vi "测试配置文件生成.vi"() -> ()   [LabVIEW 2013]
uses:
  <vilib>/Utility/config.llb/Write Key (String).vi
  <vilib>/Utility/config.llb/NI_LVConfig.lvlib
panel:
  in  "配置文件全名":path
  in  "写入至从板号":dbl=1.0 min=1.0 max=30.0
  in  "BCU合成程序全名-用于仿真器刷写":path
  in  "BMU应用程序全名":string[][](table)
  in  "更新至指定BMU号":bool
  in  "BMU应用程序全名":path
  in  "配置到全部BMU":bool
  in  "BMU个数":dbl
  in  "BCU应用程序全名-用于在线更新程序":path
  in  "充电CAN波特率":enum16{"250K", "500K"}(ring)
  in  "整车CAN波特率":enum16{"250K", "500K"}(ring)
  in  "内部CAN波特率":enum16{"250K", "500K"}(ring)
  out "取消":bool
  out "确定并启动":bool
  in  "自适就CAN卡类型":bool=TRUE
  in  "退出":bool
  in  "保存":bool
  in  "error in":errorcluster caption="错误输入"
  in  "BMU合成程序全名-用于仿真器刷写":path
  # "自动化测试配置文件生成器"
  # "将BMU应用程序全名："
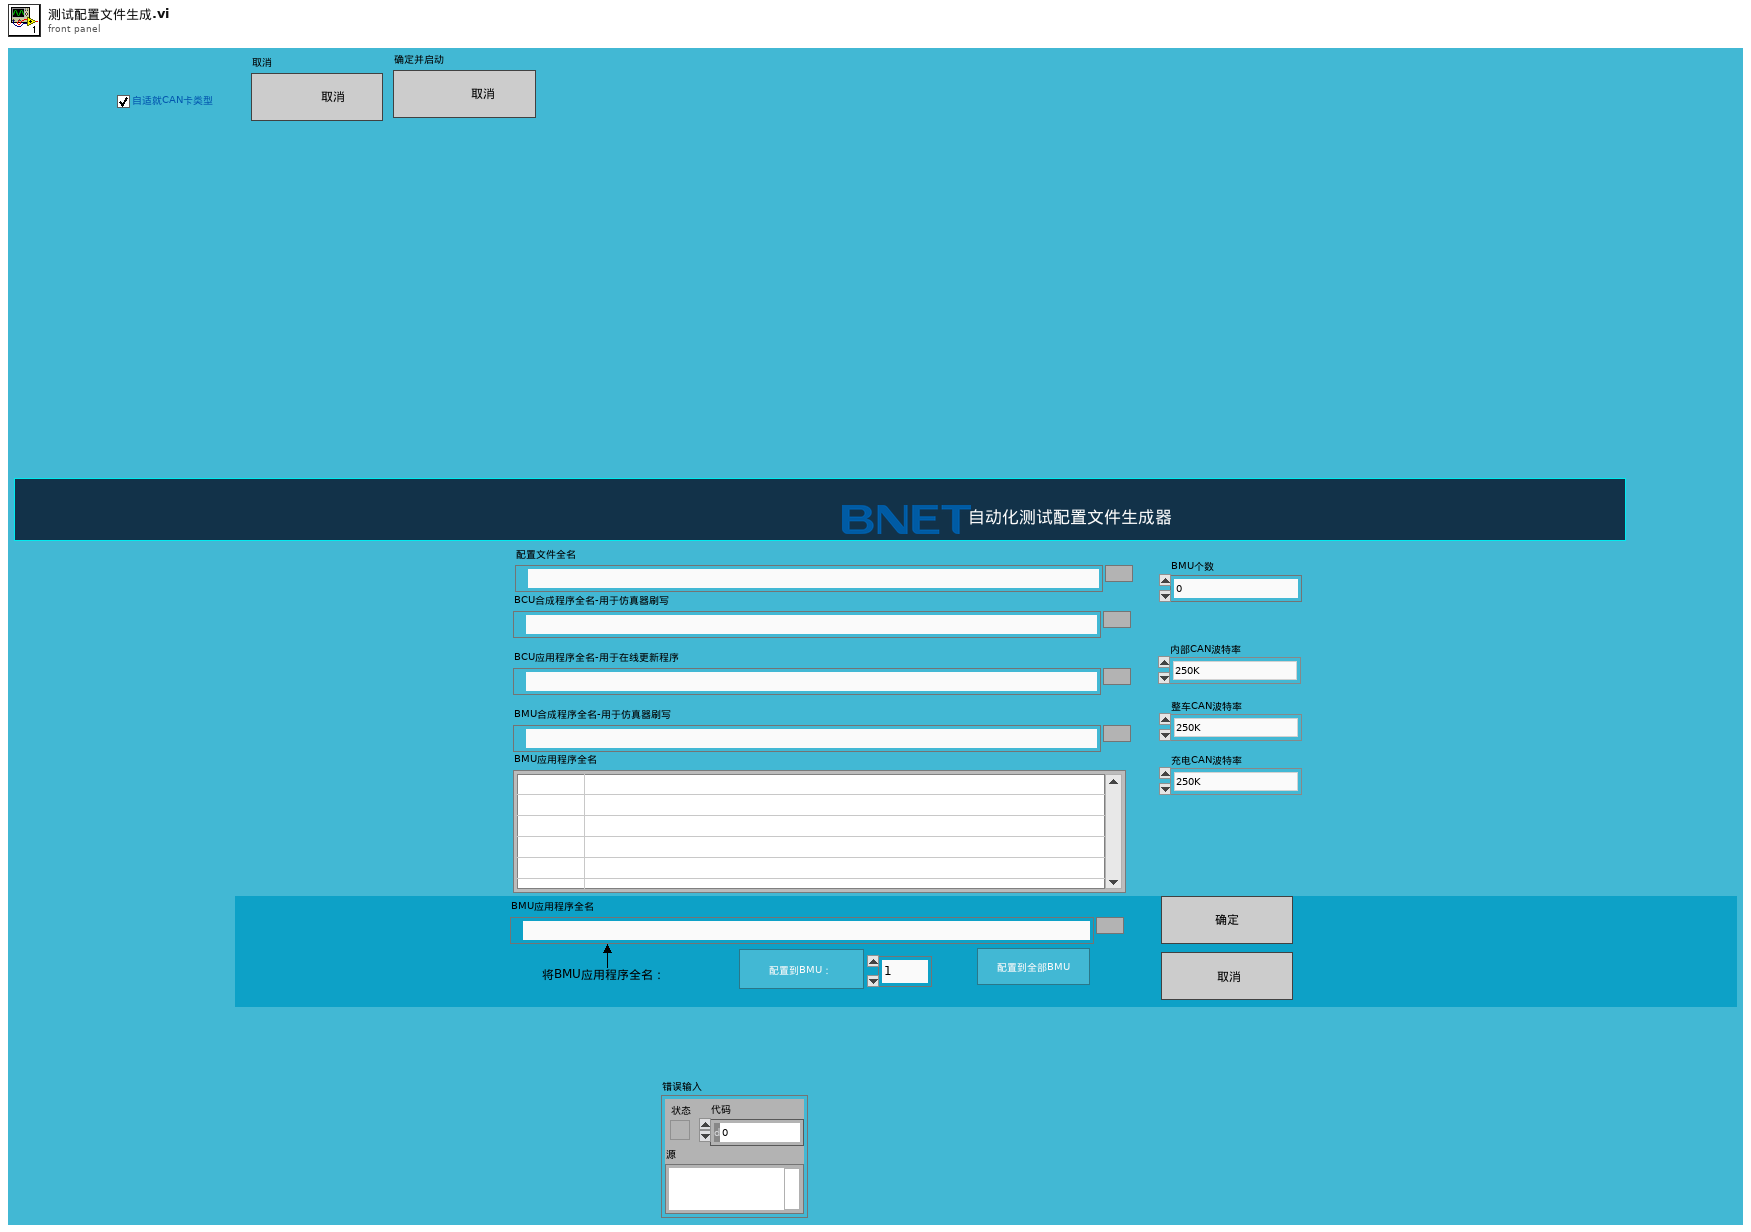
[diagram p1: front panel]
types:
  T1 = typedef "NI_LVConfig.lvlib/Config Data RefNum.ctl" = refnum<k1>
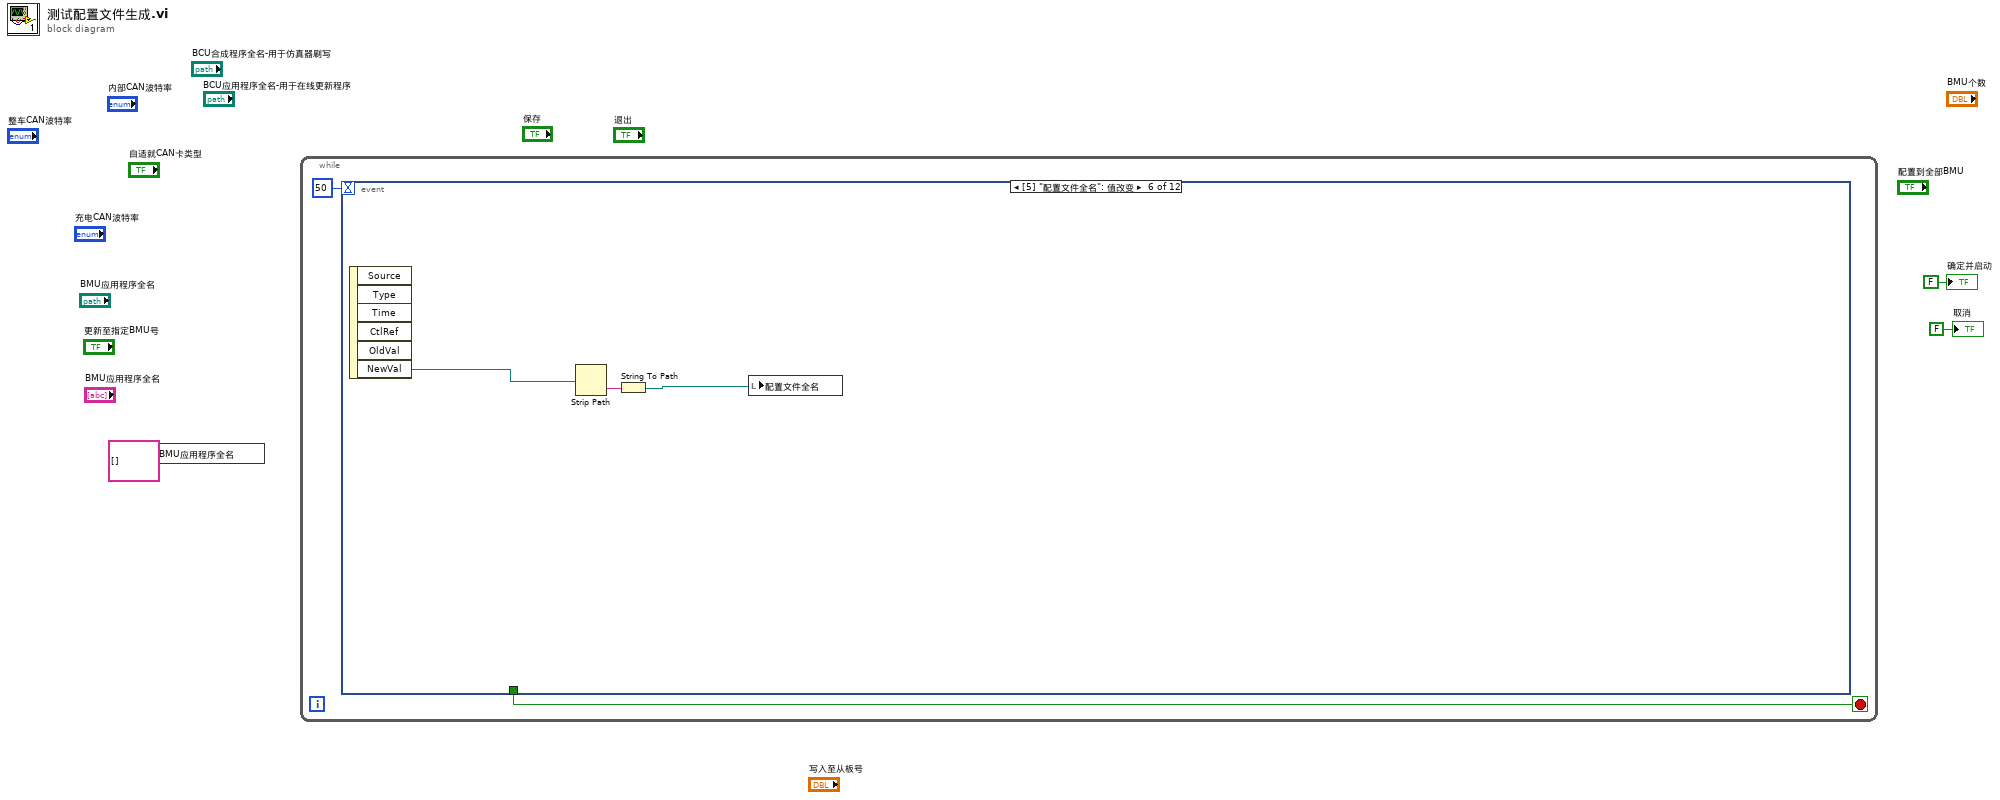
[diagram p0: block diagram]
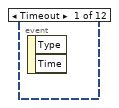
[diagram p2: hidden frame]
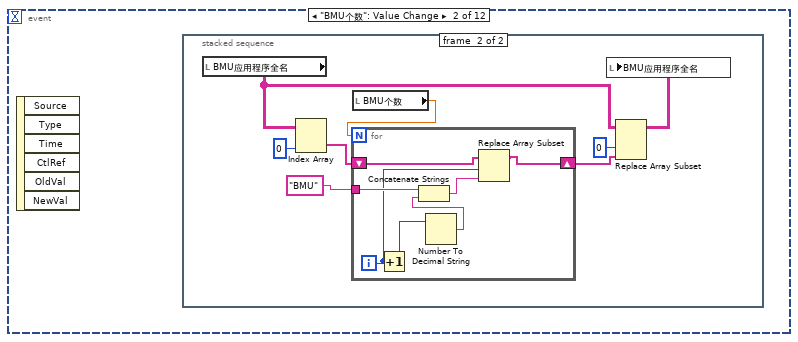
[diagram p3: hidden frame]
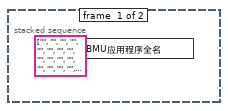
[diagram p4: hidden frame]
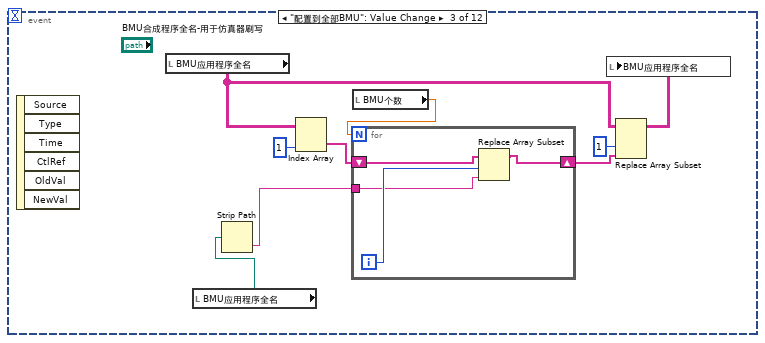
[diagram p5: hidden frame]
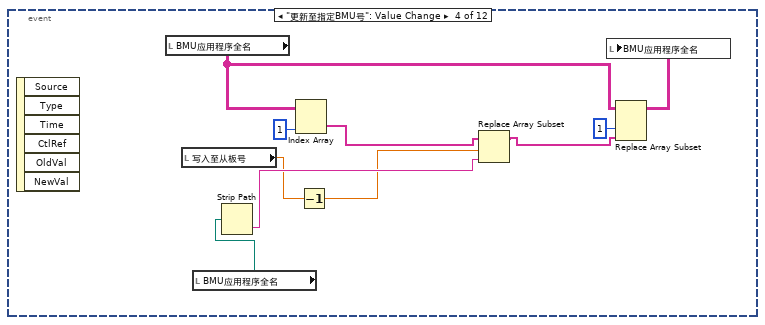
[diagram p6: hidden frame]
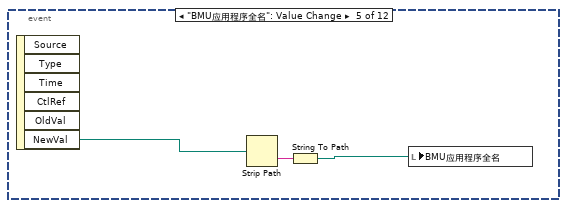
[diagram p7: hidden frame]
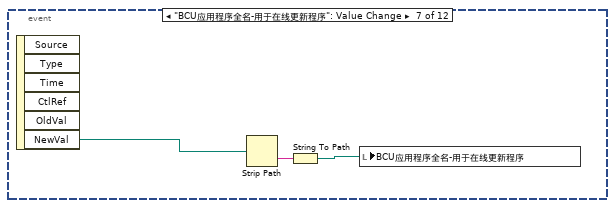
[diagram p8: hidden frame]
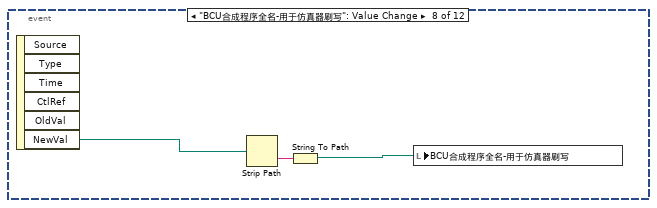
[diagram p9: hidden frame]
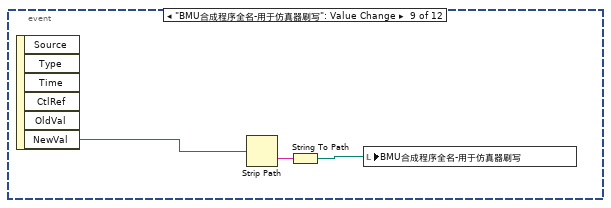
[diagram p10: hidden frame]
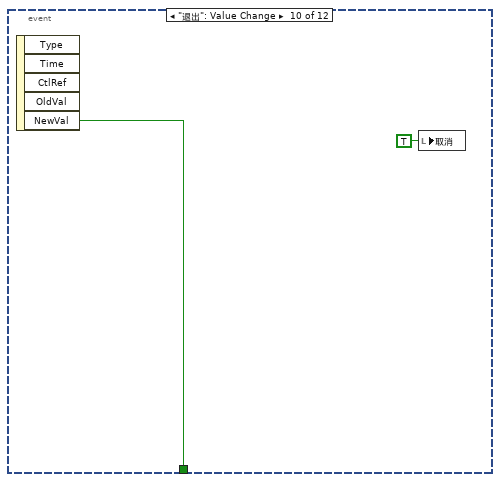
[diagram p11: hidden frame]
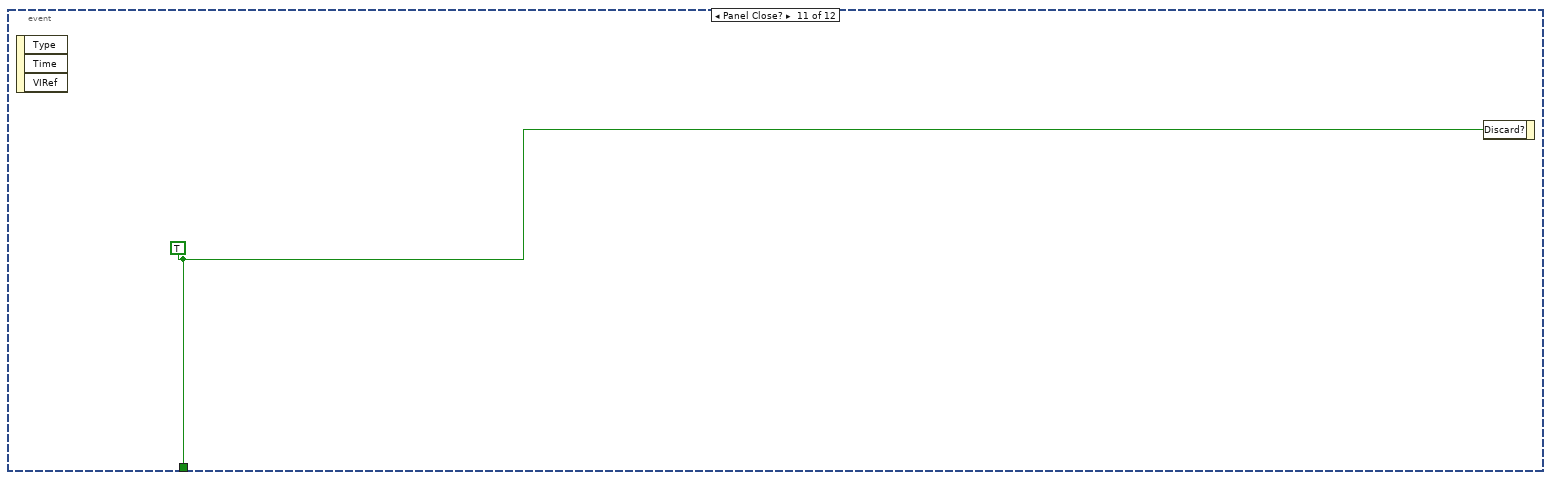
[diagram p12: hidden frame]
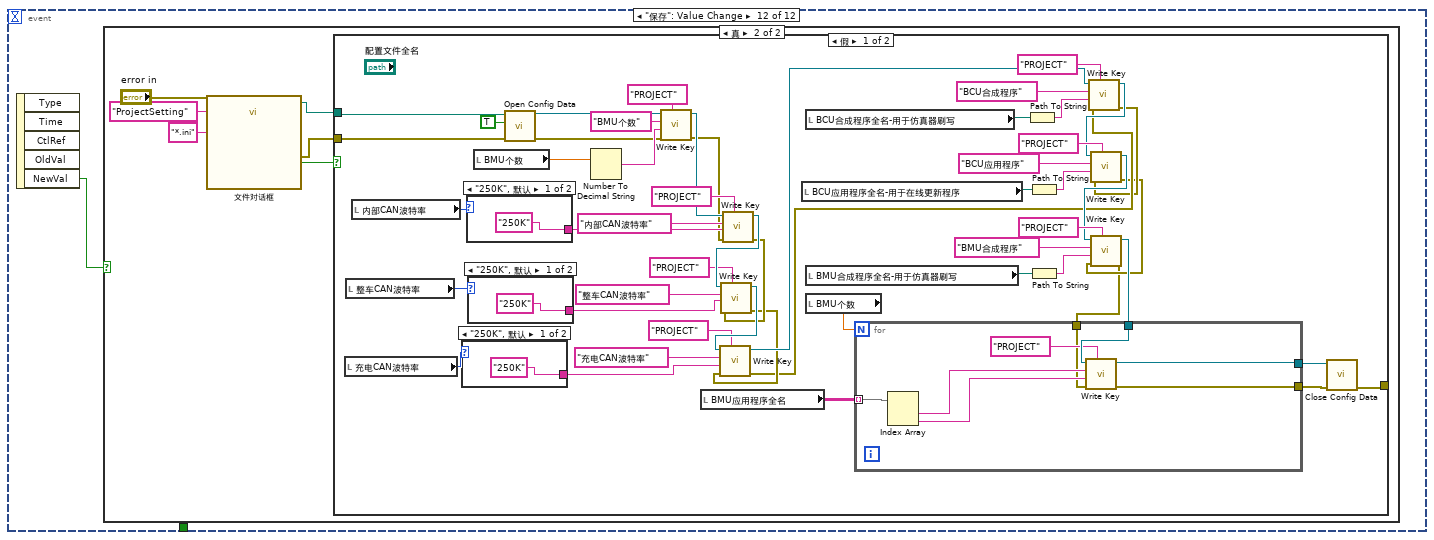
[diagram p13: hidden frame]
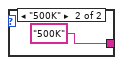
[diagram p15: hidden frame]
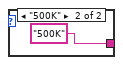
[diagram p16: hidden frame]
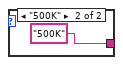
[diagram p17: hidden frame]
diagram:
  n1 = local write "BMU应用程序全名"(string[][] [] ("从板路径")) -> ()
  n2 = while {
    stop <- w5 stop-if-true
    n3 = event shown="[5] \"配置文件全名\": 值改变" {
      selector: _ -> [_ _ _ _ _ _ _ _ _ _ _ _]
      dyn-events: _ -> [_ _ _ _ _ _ _ _ _ _ _ _]
      timeout: 50 -> [_ _ _ _ _ _ _ _ _ _ _ _]
      tunnel: [_ _ _ _ _ _ _ _ _ w61 w62 _] -> w5
      event Timeout {
        n4 = event-data() -> ()  [unwired: 3 out]
      }
      event "BMU个数": Value Change {
        n5 = event-data() -> ()  [unwired: 7 out]
        n6 = stacked-sequence {
          frame #0 {
            n7 = local write "BMU应用程序全名"(string[][] [["", "", ""], ["", "", ""], ["", "", ""], ["", "", ""], ["", "", ""], ["", "", ""], ["", "", ""], ["", "", ""], ["", "", ""], ["", "", ""], ["", "", ""], ["", "", ""], ["", "", ""], ["", "", ""], ["", "", ""], ["", "", ""], ["", "", ""], ["", "", ""], ["", "", ""], ["", "", ""], ["", "", ""], ["", "", ""], ["", "", ""], ["", "", ""], ["", "", ""], ["", "", ""], ["", "", ""], ["", "", ""], ["", "", ""], ["", "", ""], ["", "", " "]] ("从板路径")) -> ()
          }
          frame #1 {
            n8 = local read "BMU应用程序全名"() -> (w10:string[][])
            n9 = Index Array(array=w10, index (col)=0 ("禁用的索引 (列)")) -> (element=w13:string[])  [unwired: 1 in]
            n10 = local read "BMU个数"() -> (w12:dbl)
            n11 = for {
              N: w12 -> [_]
              tunnel: "BMU" -> [w19]
              shift-right: [w16] -> w8
              shift-left: w13 -> [w21]
              i -> [w15]
              n12 = Increment(x=w15) -> (x+1=w20:i32)
              n13 = Number To Decimal String(number=w20) -> (decimal integer string=w18:string)  [unwired: 1 in]
              n14 = Concatenate Strings(w19, w18) -> (w17:string)
              n15 = Replace Array Subset(array=w21, new element=w17, index=w15) -> (w16:string[])
            }
            n16 = Replace Array Subset(array=w10, new element=w8, index (col)=0 ("禁用的索引 (列)")) -> (w7:string[][])  [unwired: 1 in]
            n17 = local write "BMU应用程序全名"(w7) -> ()
          }
        }
      }
      event "配置到全部BMU": Value Change {
        n18 = event-data() -> ()  [unwired: 7 out]
        n19 = local read "BMU应用程序全名"() -> (w27:string[][])
        n20 = local read "BMU应用程序全名"() -> (w23:path)
        n21 = Strip Path(path=w23) -> (name=w22:string)  [unwired: 1 out]
        n22 = Index Array(array=w27, index (col)=1 ("禁用的索引 (列)")) -> (element=w29:string[])  [unwired: 1 in]
        n23 = local read "BMU个数"() -> (w28:dbl)
        n24 = for {
          N: w28 -> [_]
          tunnel: w22 -> [w31]
          shift-right: [w33] -> w25
          shift-left: w29 -> [w34]
          i -> [w32]
          n25 = Replace Array Subset(array=w34, new element=w31, index=w32) -> (w33:string[])
        }
        n26 = Replace Array Subset(array=w27, new element=w25, index (col)=1 ("禁用的索引 (列)")) -> (w24:string[][])  [unwired: 1 in]
        n27 = local write "BMU应用程序全名"(w24) -> ()
      }
      event "更新至指定BMU号": Value Change {
        n28 = event-data() -> ()  [unwired: 7 out]
        n29 = local read "BMU应用程序全名"() -> (w42:string[][])
        n30 = local read "写入至从板号"() -> (w36:dbl)
        n31 = local read "BMU应用程序全名"() -> (w38:path)
        n32 = Strip Path(path=w38) -> (name=w37:string)  [unwired: 1 out]
        n33 = Index Array(array=w42, index (col)=1 ("禁用的索引 (列)")) -> (element=w43:string[])  [unwired: 1 in]
        n34 = Decrement(x=w36) -> (x-1=w35:dbl)
        n35 = Replace Array Subset(array=w43, new element=w37, index=w35) -> (w40:string[])
        n36 = Replace Array Subset(array=w42, new element=w40, index (col)=1 ("禁用的索引 (列)")) -> (w39:string[][])  [unwired: 1 in]
        n37 = local write "BMU应用程序全名"(w39) -> ()
      }
      event "BMU应用程序全名": Value Change {
        n38 = event-data() -> ("NewVal"=w47:path)  [unwired: 6 out]
        n39 = Strip Path(path=w47) -> (name=w46:string)  [unwired: 1 out]
        n40 = String To Path(string=w46) -> (path=w45:path)
        n41 = local write "BMU应用程序全名"(w45) -> ()
      }
      event "配置文件全名": Value Change {
        n42 = event-data() -> ("NewVal"=w50:path)  [unwired: 6 out]
        n43 = Strip Path(path=w50) -> (name=w49:string)  [unwired: 1 out]
        n44 = String To Path(string=w49) -> (path=w48:path)
        n45 = local write "配置文件全名"(w48) -> ()
      }
      event "BCU应用程序全名-用于在线更新程序": Value Change {
        n46 = event-data() -> ("NewVal"=w53:path)  [unwired: 6 out]
        n47 = Strip Path(path=w53) -> (name=w52:string)  [unwired: 1 out]
        n48 = String To Path(string=w52) -> (path=w51:path)
        n49 = local write "BCU应用程序全名-用于在线更新程序"(w51) -> ()
      }
      event "BCU合成程序全名-用于仿真器刷写": Value Change {
        n50 = event-data() -> ("NewVal"=w56:path)  [unwired: 6 out]
        n51 = Strip Path(path=w56) -> (name=w55:string)  [unwired: 1 out]
        n52 = String To Path(string=w55) -> (path=w54:path)
        n53 = local write "BCU合成程序全名-用于仿真器刷写"(w54) -> ()
      }
      event "BMU合成程序全名-用于仿真器刷写": Value Change {
        n54 = event-data() -> ("NewVal"=w59:path)  [unwired: 6 out]
        n55 = Strip Path(path=w59) -> (name=w58:string)  [unwired: 1 out]
        n56 = String To Path(string=w58) -> (path=w57:path)
        n57 = local write "BMU合成程序全名-用于仿真器刷写"(w57) -> ()
      }
      event "退出": Value Change {
        n58 = event-data() -> ("NewVal"=w61:bool)  [unwired: 5 out]
        n59 = local write "取消"(TRUE ("取消")) -> ()
      }
      event Panel Close? {
        w62 = TRUE ("NewVal")
        n60 = event-data() -> ()  [unwired: 4 out]
        n61 = event-data("Discard?"=w62) -> ()  [unwired: 1 in, 1 out]
      }
      event "保存": Value Change {
        n62 = event-data() -> ("NewVal"=w63:bool)  [unwired: 5 out]
        n63 = case shown="真" w63 {
          frame False {
          }
          frame True {
            n64 = call "文件对话框"("default name"="ProjectSetting", "error in"="error in", "pattern (all files)"="*.ini") -> ("selected path"=w68:path, "cancelled"=w69:bool, "error out"=w64:errorcluster)  [unwired: 9 in, 1 out]
            n65 = case shown="假" w69 {
              tunnel: w68 -> [w121 _]
              tunnel: w64 -> [w80 _]
              tunnel: [w70 _] -> _
              frame False {
                n66 = local read "充电CAN波特率"() -> (w102:enum16{"250K", "500K"})
                n67 = local read "整车CAN波特率"() -> (w105:enum16{"250K", "500K"})
                n68 = local read "内部CAN波特率"() -> (w103:enum16{"250K", "500K"})
                n69 = case shown="\"250K\", 默认" w102 {
                  tunnel: ["250K" ("key") "500K" ("key")] -> w82
                  frame "250K", Default {
                  }
                  frame "500K" {
                  }
                }
                n70 = case shown="\"250K\", 默认" w103 {
                  tunnel: ["250K" ("key") "500K" ("key")] -> w81
                  frame "250K", Default {
                  }
                  frame "500K" {
                  }
                }
                n71 = case shown="\"250K\", 默认" w105 {
                  tunnel: ["250K" ("key") "500K" ("key")] -> w104
                  frame "250K", Default {
                  }
                  frame "500K" {
                  }
                }
                n72 = local read "BMU个数"() -> (w116:dbl)
                n73 = call <vilib>:"Open Config Data.vi"("error in (no error)"=w80, "create file if necessary (T)"=TRUE, "configuration file path"=w121) -> ("error out"=w79:errorcluster, "refnum"=w119:T1)  [unwired: 6 in, 1 out]
                n74 = Number To Decimal String(number=w116) -> (decimal integer string=w115:string)  [unwired: 1 in]
                n75 = call-poly <vilib>:"Write Key.vi"("section"="PROJECT", "error in (no error)"=w79, "value"=w115, "key"="BMU个数", "refnum"=w119) -> ("error out"=w78:errorcluster, "refnum out"=w114:T1)  [unwired: 4 in, 1 out]
                n76 = local read "BMU应用程序全名"() -> (w84:string[][])
                n77 = call-poly <vilib>:"Write Key.vi"("section"="PROJECT", "error in (no error)"=w78, "value"=w81, "key"="内部CAN波特率", "refnum"=w114) -> ("error out"=w77:errorcluster, "refnum out"=w110:T1)  [unwired: 4 in, 1 out]
                n78 = call-poly <vilib>:"Write Key.vi"("section"="PROJECT", "error in (no error)"=w77, "value"=w104, "key"="整车CAN波特率", "refnum"=w110) -> ("error out"=w76:errorcluster, "refnum out"=w109:T1)  [unwired: 4 in, 1 out]
                n79 = call-poly <vilib>:"Write Key.vi"("section"="PROJECT", "error in (no error)"=w76, "value"=w82, "key"="充电CAN波特率", "refnum"=w109) -> ("error out"=w75:errorcluster, "refnum out"=w99:T1)  [unwired: 4 in, 1 out]
                n80 = local read "BCU应用程序全名-用于在线更新程序"() -> (w95:path)
                n81 = local read "BCU合成程序全名-用于仿真器刷写"() -> (w98:path)
                n82 = local read "BMU合成程序全名-用于仿真器刷写"() -> (w89:path)
                n83 = local read "BMU个数"() -> (w85:dbl)
                n84 = Path To String(path=w98) -> (string=w97:string)
                n85 = Path To String(path=w95) -> (string=w96:string)
                n86 = Path To String(path=w89) -> (string=w88:string)
                n87 = call-poly <vilib>:"Write Key.vi"("section"="PROJECT", "error in (no error)"=w75, "value"=w97, "key"="BCU合成程序", "refnum"=w99) -> ("error out"=w74:errorcluster, "refnum out"=w92:T1)  [unwired: 4 in, 1 out]
                n88 = call-poly <vilib>:"Write Key.vi"("section"="PROJECT", "error in (no error)"=w74, "value"=w96, "key"="BCU应用程序", "refnum"=w92) -> ("error out"=w73:errorcluster, "refnum out"=w87:T1)  [unwired: 4 in, 1 out]
                n89 = call-poly <vilib>:"Write Key.vi"("section"="PROJECT", "error in (no error)"=w73, "value"=w88, "key"="BMU合成程序", "refnum"=w87) -> ("error out"=w72:errorcluster, "refnum out"=w86:T1)  [unwired: 4 in, 1 out]
                n90 = for {
                  N: w85 -> [_]
                  tunnel: w86 -> [w129]
                  tunnel: w84 -> [w128] mode=indexing
                  tunnel: [w125] -> w83
                  tunnel: w72 -> [w123]
                  tunnel: [w122] -> w71
                  n91 = Index Array(array=w128) -> (element #1=w127:string, element #2=w126:string)  [unwired: 2 in]
                  n92 = call-poly <vilib>:"Write Key.vi"("section"="PROJECT", "error in (no error)"=w123, "value"=w126, "key"=w127, "refnum"=w129) -> ("error out"=w122:errorcluster, "refnum out"=w125:T1)  [unwired: 4 in, 1 out]
                }
                n93 = call <vilib>:"Close Config Data.vi"("error in (no error)"=w71, "refnum"=w83) -> ("error out"=w70:errorcluster)  [unwired: 8 in, 1 out]
              }
              frame True {
              }
            }
          }
        }
      }
    }
  }
  "确定并启动" <- FALSE ("确定并启动")
  "取消" <- FALSE ("取消")
